vi "Sys Config-format and values.vi"(0 "System Config":T4={"XY Stage"={"COM port"="", "XY stage available"=FALSE}, "DAQ FPGA"={"Ref"=refnum, "Target"="RIO0", "Clock Freq (MHz) "=200.0, "input card type"=enum."AC Card", "Samples Wait after Trigger"=5080, "AOD fill"=4900, "StartupDelay"=0, "Slip Cycle (clock cycles)"=600000, "Add Cycle"=TRUE}, "Control system"={"Ethernet opened"=FALSE, "Ethernet Port"=3, "Ctrl FPGA available"=FALSE, "Ctrl FPGA Clock (MHz)"=240.0, "Ctrl system MAC address"="", "Control system.Network adapter name"="", "AOD 1 Amplitude"=0, "AOD 2 Amplitude"=0, "AOD 3 Amplitude"=0, "AOD 4 Amplitude"=0, "Data Time Interval (ns)"=0.0, "T0 (ns)"=0.0, "Ta (ns)"=0.0}, "Encoder"={"IP address"="224.0.1.103", "Port"=7000, "Encoder available"=FALSE, "Wheel radius (cm)"=16.0}, "DAQmx Chan"={"Pockels AO"="", "Hard shutter AO"="", "PMT AOs"="", "Power meter AI"=""}, "Computer MAC address"="", "Cam VidRec"={"DO flag-Video record"="", "DO flag-Trial start"="", "VidRec available"=FALSE}, "Externalise Triggers"=FALSE, "Laser wavelength (nm)"=920.0} {"Laser wavelength (nm)" min=800.0 max=1080.0 step=1.0; "Encoder"."Wheel radius (cm)" format="%#_13g"; "Control system"."Ctrl FPGA Clock (MHz)" min=80.0 max=500.0 step=1.0; "Control system"."Data Time Interval (ns)" min=0.0 max=2048.0 step=1.0; "Control system"."Ta (ns)" min=0.0 max=2048.0 step=1.0; "Control system"."T0 (ns)" min=0.0 max=2048.0 step=1.0; "Control system"."AOD 4 Amplitude" min=0 max=2048 step=1; "Control system"."AOD 3 Amplitude" min=0 max=2048 step=1; "Control system"."AOD 2 Amplitude" min=0 max=2048 step=1; "Control system"."AOD 1 Amplitude" min=0 max=2048 step=1}) -> (14 "Keys setup.DBL":T2=[{"key"="Control FPGA.Clock Freq (MHz)", "Save?"=TRUE, "Default"=240.0}, {"key"="DAQ FPGA.Clock Freq (MHz)", "Save?"=TRUE, "Default"=240.0}], 15 "Values.DBL":dbl[](array[numeric]), 16 "Keys setup.String":T3=[{"key"="Control FPGA.MAC address", "Save?"=TRUE, "Default"="AABBCCDDEEFF"}, {"key"="DAQ FPGA.Target", "Save?"=TRUE, "Default"="RIO0"}, {"key"="XY Stage.COM port", "Save?"=TRUE, "Default"="COM7"}, {"key"="DAQmx Chan.Pockels Control", "Save?"=TRUE, "Default"=""}, {"key"="DAQmx Chan.Hard Shutter", "Save?"=TRUE, "Default"=""}, {"key"="DAQmx Chan.PMT 1", "Save?"=TRUE, "Default"=""}, {"key"="DAQmx Chan.PMT 2", "Save?"=TRUE, "Default"=""}, {"key"="DAQmx Chan.Encoder Trigger", "Save?"=TRUE, "Default"=""}, {"key"="DAQmx Chan.Optional Trigger 1", "Save?"=TRUE, "Default"=""}, {"key"="DAQmx Chan.Optional Trigger 2", "Save?"=TRUE, "Default"=""}, {"key"="DAQmx Chan.Optional Trigger 3", "Save?"=TRUE, "Default"=""}], 17 "Values.Strings":string[](array[string]), 18 "Keys setup.Boolean":T1, 19 "Values.Boolean":bool[](array[boolean]))   [LabVIEW 2013]
uses:
  Typedefs/Sys Configuration.ctl
  Typedefs/XY Stage config cluster.ctl
  Typedefs/DAQ FPGA config cluster.ctl
  RIG-SPECIFIC FILES/FPGA Refs/FPGA Ref.ctl
  <vilib>/userdefined/High Color/nirio_resource_hc.ctl
  Typedefs/FPGA input type AC-DC.ctl
  Typedefs/CTRL system config cluster.ctl
  Typedefs/Encoder config cluster.ctl
  Typedefs/DAQmx physical channels cluster.ctl
  Typedefs/Cam VidRec HW config setup cluster.ctl
  Typedefs/Ini file interface (String).ctl
  Typedefs/Ini file interface (DBL).ctl
  Typedefs/Ini file interface (Boolean).ctl
panel:
  # "NOTES:\n1. \"Control FPGA.Ethernet port\" is detected automatically. It is not saved/loaded from file.\n2. \"Control FPGA.Ethernet Opened\" is detected automatically. It is not saved/loaded from file."
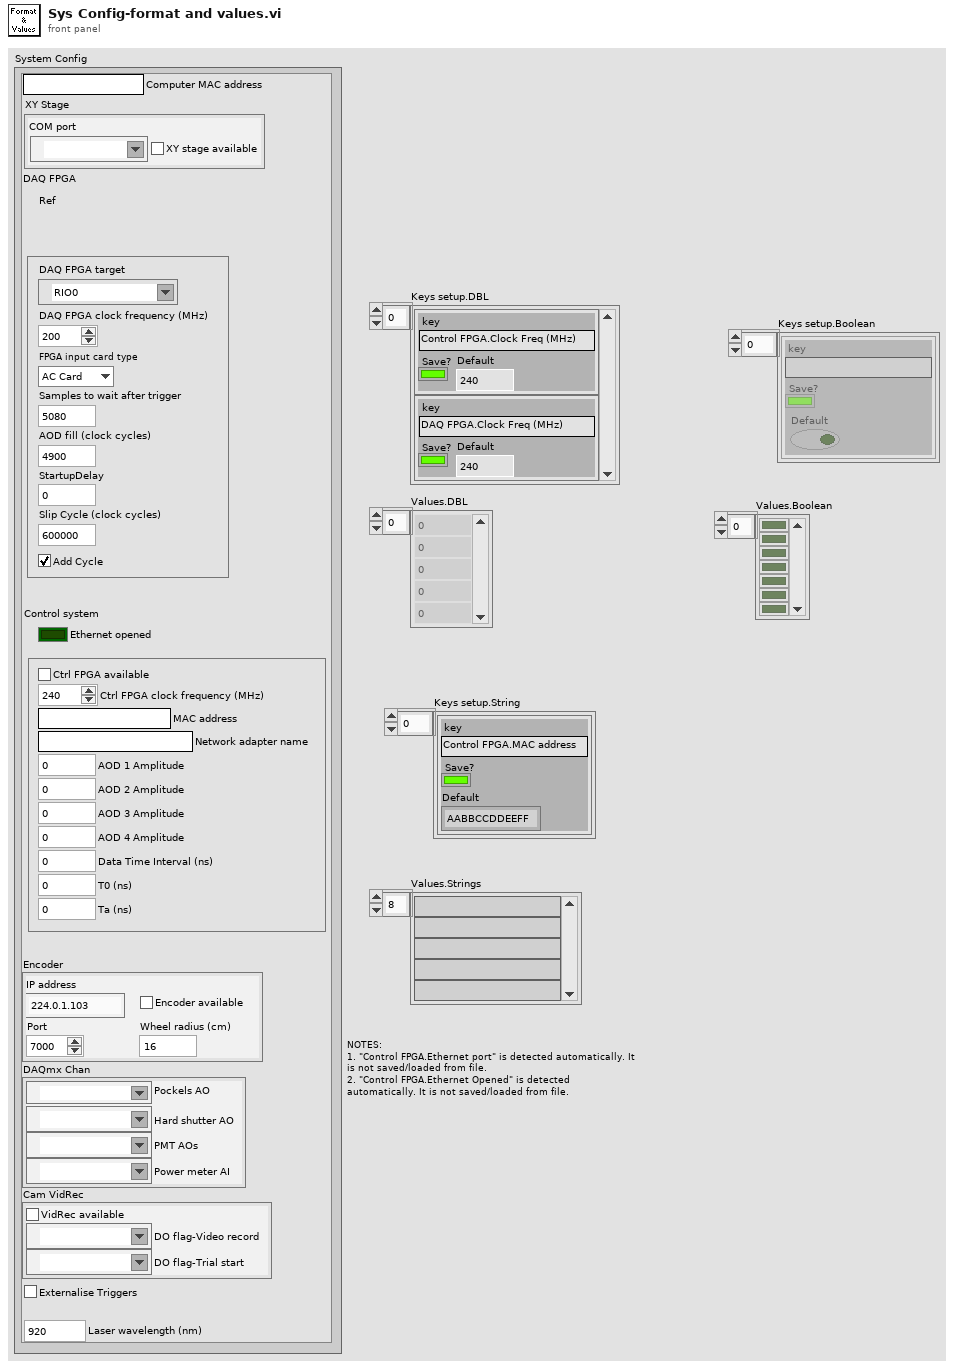
[diagram p1: front panel]
types:
  T1 = typedef "Ini file interface (Boolean).ctl" = cluster{"key":string, "Save?":bool, "Default":bool}[]
  T2 = typedef "Ini file interface (DBL).ctl" = cluster{"key":string, "Save?":bool, "Default":dbl}[]
  T3 = typedef "Ini file interface (String).ctl" = cluster{"key":string, "Save?":bool, "Default":string}[]
  T4 = typedef "Sys Configuration.ctl" = cluster{"XY Stage":T5, "DAQ FPGA":T6, "Control system":T10, "Encoder":T11, "DAQmx Chan":T12, "Computer MAC address":string, "Cam VidRec":T13, "Externalise Triggers":bool, "Laser wavelength (nm)":dbl}
  T5 = typedef "XY Stage config cluster.ctl" = cluster{"COM port":refnum<visa-resource-name>, "XY stage available":bool}
  T6 = typedef "DAQ FPGA config cluster.ctl" = cluster{"Ref":T7, "Target":T8, "Clock Freq (MHz) ":dbl, "input card type":T9, "Samples Wait after Trigger":u16, "AOD fill":u16, "StartupDelay":i32, "Slip Cycle (clock cycles)":u32, "Add Cycle":bool}
  T7 = typedef "FPGA Ref.ctl" = refnum<k20>
  T8 = typedef "nirio_resource_hc.ctl" = tag
  T9 = typedef "FPGA input type AC-DC.ctl" = enum16{"AC Card", "DC Card"}
  T10 = typedef "CTRL system config cluster.ctl" = cluster{"Ethernet opened":bool, "Ethernet Port":u32, "Ctrl FPGA available":bool, "Ctrl FPGA Clock (MHz)":dbl, "Ctrl system MAC address":string, "Control system.Network adapter name":string, "AOD 1 Amplitude":i16, "AOD 2 Amplitude":i16, "AOD 3 Amplitude":i16, "AOD 4 Amplitude":i16, "Data Time Interval (ns)":dbl, "T0 (ns)":dbl, "Ta (ns)":dbl}
  T11 = typedef "Encoder config cluster.ctl" = cluster{"IP address":string, "Port":u16, "Encoder available":bool, "Wheel radius (cm)":dbl}
  T12 = typedef "DAQmx physical channels cluster.ctl" = cluster{"Pockels AO":tag, "Hard shutter AO":tag, "PMT AOs":tag, "Power meter AI":tag}
  T13 = typedef "Cam VidRec HW config setup cluster.ctl" = cluster{"DO flag-Video record":tag, "DO flag-Trial start":tag, "VidRec available":bool}
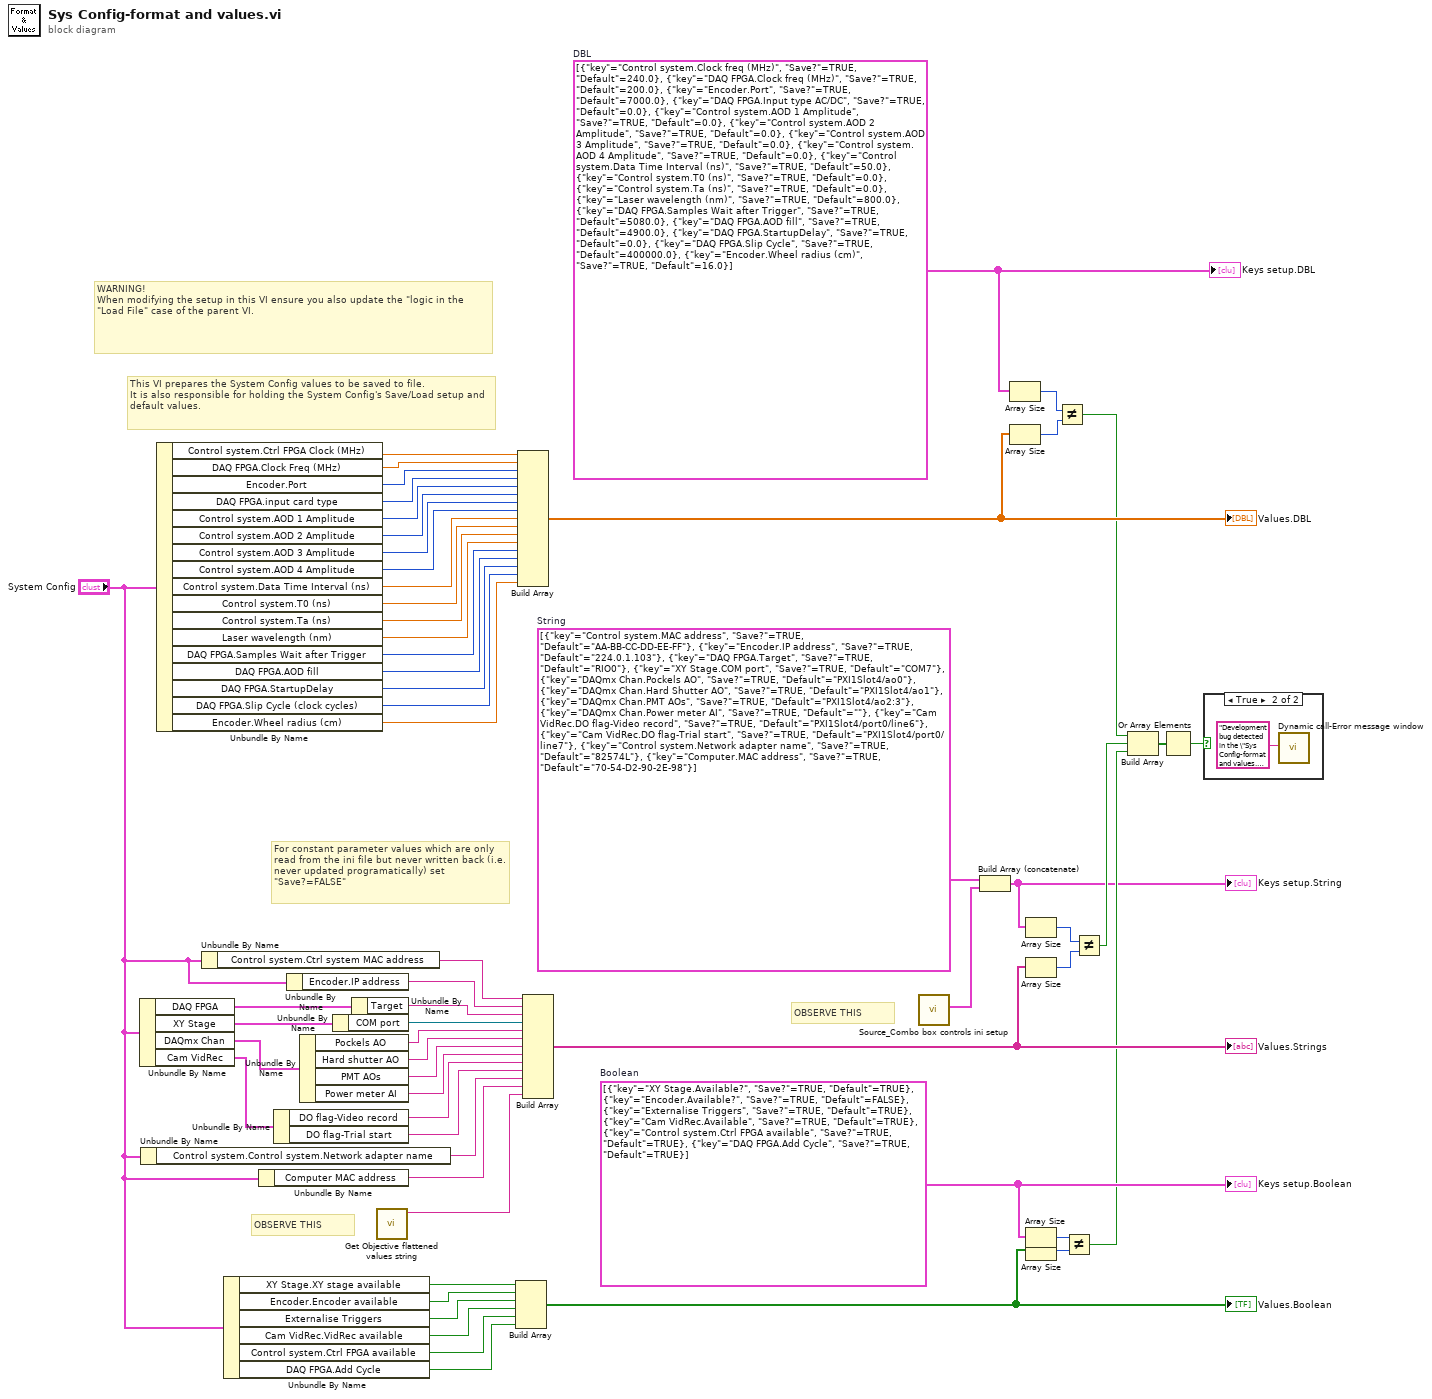
[diagram p0: block diagram]
diagram:
  w48 = T1 [{"key"="XY Stage.Available?", "Save?"=TRUE, "Default"=TRUE}, {"key"="Encoder.Available?", "Save?"=TRUE, "Default"=FALSE}, {"key"="Externalise Triggers", "Save?"=TRUE, "Default"=TRUE}, {"key"="Cam VidRec.Available", "Save?"=TRUE, "Default"=TRUE}, {"key"="Control system.Ctrl FPGA available", "Save?"=TRUE, "Default"=TRUE}, {"key"="DAQ FPGA.Add Cycle", "Save?"=TRUE, "Default"=TRUE}]  # Boolean
  w6 = T3 [{"key"="Control system.MAC address", "Save?"=TRUE, "Default"="AA-BB-CC-DD-EE-FF"}, {"key"="Encoder.IP address", "Save?"=TRUE, "Default"="224.0.1.103"}, {"key"="DAQ FPGA.Target", "Save?"=TRUE, "Default"="RIO0"}, {"key"="XY Stage.COM port", "Save?"=TRUE, "Default"="COM7"}, {"key"="DAQmx Chan.Pockels AO", "Save?"=TRUE, "Default"="PXI1Slot4/ao0"}, {"key"="DAQmx Chan.Hard Shutter AO", "Save?"=TRUE, "Default"="PXI1Slot4/ao1"}, {"key"="DAQmx Chan.PMT AOs", "Save?"=TRUE, "Default"="PXI1Slot4/ao2:3"}, {"key"="DAQmx Chan.Power meter AI", "Save?"=TRUE, "Default"=""}, {"key"="Cam VidRec.DO flag-Video record", "Save?"=TRUE, "Default"="PXI1Slot4/port0/line6"}, {"key"="Cam VidRec.DO flag-Trial start", "Save?"=TRUE, "Default"="PXI1Slot4/port0/line7"}, {"key"="Control system.Network adapter name", "Save?"=TRUE, "Default"="82574L"}, {"key"="Computer.MAC address", "Save?"=TRUE, "Default"="70-54-D2-90-2E-98"}]  # String
  w51 = T2 [{"key"="Control system.Clock freq (MHz)", "Save?"=TRUE, "Default"=240.0}, {"key"="DAQ FPGA.Clock freq (MHz)", "Save?"=TRUE, "Default"=200.0}, {"key"="Encoder.Port", "Save?"=TRUE, "Default"=7000.0}, {"key"="DAQ FPGA.Input type AC/DC", "Save?"=TRUE, "Default"=0.0}, {"key"="Control system.AOD 1 Amplitude", "Save?"=TRUE, "Default"=0.0}, {"key"="Control system.AOD 2 Amplitude", "Save?"=TRUE, "Default"=0.0}, {"key"="Control system.AOD 3 Amplitude", "Save?"=TRUE, "Default"=0.0}, {"key"="Control system.AOD 4 Amplitude", "Save?"=TRUE, "Default"=0.0}, {"key"="Control system.Data Time Interval (ns)", "Save?"=TRUE, "Default"=50.0}, {"key"="Control system.T0 (ns)", "Save?"=TRUE, "Default"=0.0}, {"key"="Control system.Ta (ns)", "Save?"=TRUE, "Default"=0.0}, {"key"="Laser wavelength (nm)", "Save?"=TRUE, "Default"=800.0}, {"key"="DAQ FPGA.Samples Wait after Trigger", "Save?"=TRUE, "Default"=5080.0}, {"key"="DAQ FPGA.AOD fill", "Save?"=TRUE, "Default"=4900.0}, {"key"="DAQ FPGA.StartupDelay", "Save?"=TRUE, "Default"=0.0}, {"key"="DAQ FPGA.Slip Cycle", "Save?"=TRUE, "Default"=400000.0}, {"key"="Encoder.Wheel radius (cm)", "Save?"=TRUE, "Default"=16.0}]  # DBL
  # "OBSERVE THIS"
  # "OBSERVE THIS"
  # "WARNING!\nWhen modifying the setup in this VI ensure you also update the \"logic in the \"Load File\" case of the parent VI."
  # "For constant parameter values which are only read from the ini file but never written back (i.e. never updated programatically) set \"Save?=FALSE\""
  # "This VI prepares the System Config values to be saved to file.\nIt is also responsible for holding the System Config's Save/Load setup and default values."
  n1 = Unbundle By Name("System Config") -> ("DAQ FPGA"=w55:T6, "XY Stage"=w57:T5, "DAQmx Chan"=w60:T12, "Cam VidRec"=w21:T13)
  n2 = Unbundle By Name("System Config") -> ("Control system.Control system.Network adapter name"=w31:string)
  n3 = Unbundle By Name("System Config") -> ("Control system.Ctrl FPGA Clock (MHz)"=w52:dbl, "DAQ FPGA.Clock Freq (MHz)"=w34:dbl, "Encoder.Port"=w33:u16, "DAQ FPGA.input card type"=w32:T9, "Control system.AOD 1 Amplitude"=w20:i16, "Control system.AOD 2 Amplitude"=w19:i16, "Control system.AOD 3 Amplitude"=w18:i16, "Control system.AOD 4 Amplitude"=w17:i16, "Control system.Data Time Interval (ns)"=w15:dbl, "Control system.T0 (ns)"=w14:dbl, "Control system.Ta (ns)"=w13:dbl, "Laser wavelength (nm)"=w12:dbl, "DAQ FPGA.Samples Wait after Trigger"=w11:u16, "DAQ FPGA.AOD fill"=w10:u16, "DAQ FPGA.StartupDelay"=w9:i32, "DAQ FPGA.Slip Cycle (clock cycles)"=w8:u32, "Encoder.Wheel radius (cm)"=w1:dbl)
  n4 = Unbundle By Name("System Config") -> ("Control system.Ctrl system MAC address"=w36:string)
  n5 = Unbundle By Name("System Config") -> ("XY Stage.XY stage available"=w28:bool, "Encoder.Encoder available"=w29:bool, "Externalise Triggers"=w25:bool, "Cam VidRec.VidRec available"=w24:bool, "Control system.Ctrl FPGA available"=w16:bool, "DAQ FPGA.Add Cycle"=w7:bool)
  n6 = Unbundle By Name("System Config") -> ("Computer MAC address"=w30:string)
  n7 = Unbundle By Name(w21) -> ("DO flag-Video record"=w23:tag, "DO flag-Trial start"=w22:tag)
  n8 = Unbundle By Name("System Config") -> ("Encoder.IP address"=w35:string)
  n9 = Unbundle By Name(w60) -> ("Pockels AO"=w56:tag, "Hard shutter AO"=w59:tag, "PMT AOs"=w58:tag, "Power meter AI"=w2:tag)
  n10 = Unbundle By Name(w57) -> ("COM port"=w54:refnum<visa-resource-name>)
  n11 = Unbundle By Name(w55) -> ("Target"=w53:T8)
  n12 = call "Get Objective flattened values string.vi"() -> ("\"Objective\" control's flattened values string"=w3:string)  [unwired: 9 in, 2 out]
  n13 = Build Array(w28, w29, w25, w24, w16, w7) -> (w26:bool[])
  "Values.Boolean" <- w26
  n14 = Build Array(w52, w34, w33, w32, w20, w19, w18, w17, w15, w14, w13, w12, w11, w10, w9, w8, w1) -> (w49:dbl[])
  "Values.DBL" <- w49
  n15 = Build Array(w36, w35, w53, w54, w56, w59, w58, w2, w23, w22, w31, w30, w3) -> (w50:string[])
  "Values.Strings" <- w50
  n16 = call "Source_Combo box controls ini setup.vi"() -> ("Keys setup"=w4:T3)  [unwired: 10 in, 1 out]
  n17 = Build Array (concatenate)(w6, w4) -> (w5:T3)
  "Keys setup.String" <- w5
  n18 = Array Size(array=w51) -> (size(s)=w45:i32)
  n19 = Array Size(array=w49) -> (size(s)=w44:i32)
  n20 = Array Size(array=w5) -> (size(s)=w47:i32)
  n21 = Array Size(array=w50) -> (size(s)=w46:i32)
  n22 = Array Size(array=w48) -> (size(s)=w43:i32)
  n23 = Array Size(array=w26) -> (size(s)=w42:i32)
  n24 = Not Equal?(x=w45, y=w44) -> (x != y?=w38:bool)
  n25 = Not Equal?(x=w43, y=w42) -> (x != y?=w40:bool)
  n26 = Not Equal?(x=w47, y=w46) -> (x != y?=w37:bool)
  n27 = Build Array(w38, w37, w40) -> (w41:bool[])
  n28 = Or Array Elements(Boolean array=w41) -> (logical OR=w39:bool)
  n29 = case shown="True" w39 {
    frame False {
    }
    frame True {
      n30 = call "Dynamic call-Error message window.vi"("Error Message"="Development bug detected in the \"Sys Config-format and values.vi\".\nPlease correct the set up in this VI.") -> ()  [unwired: 10 in, 1 out]
    }
  }
  "Keys setup.DBL" <- w51
  "Keys setup.Boolean" <- w48
